vi "Move Negative Limit.vi"(8 "error in (no error)":errorcluster, 10 "Port In":T1, 11 "Controller #":string) -> (0 "error out":errorcluster, 2 "Port Out":T1)   [LabVIEW 2021]
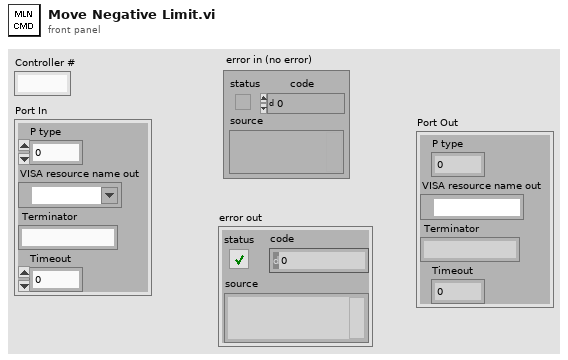
[diagram p1: front panel]
types:
  T1 = cluster{"P type":u16, "VISA resource name out":refnum<visa-resource-name>, " Terminator":string, "Timeout":i32}
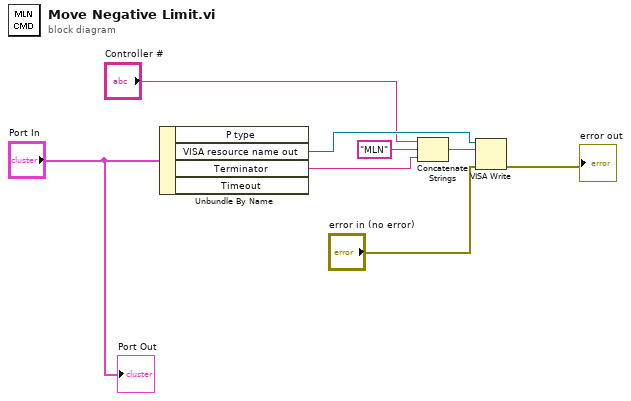
[diagram p0: block diagram]
diagram:
  n1 = Unbundle By Name("Port In") -> ("VISA resource name out"=w4:refnum<visa-resource-name>, "Terminator"=w5:string)  [unwired: 2 out]
  n2 = Concatenate Strings("Controller #", "MLN" ("string"), w5) -> (w7:string)
  n3 = VISA Write(VISA resource name=w4, write buffer=w7, error in (no error)="error in (no error)") -> (error out=→"error out":errorcluster)  [unwired: 2 out]
  "Port Out" <- "Port In"
